vi "data to acc_gyro.vi"(0 "byte array":u8[](array[numeric]), 1 "gyro range (deg/s)":dbl=250.0, 2 "accel range (m/s2)":dbl=8.0) -> (3 "acc gyro data":T1)   [LabVIEW 2012]
uses:
  acc_gyro_data.ctl
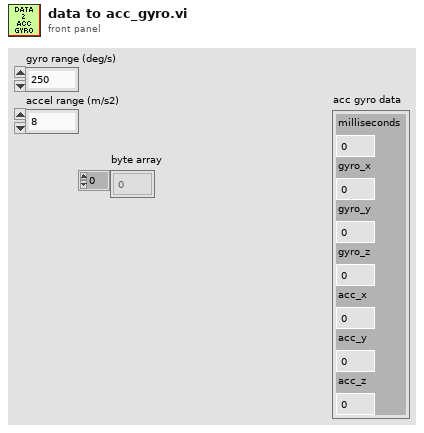
[diagram p1: front panel]
types:
  T1 = typedef "acc_gyro_data.ctl" = cluster{"milliseconds":u64, "gyro_x":dbl, "gyro_y":dbl, "gyro_z":dbl, "acc_x":dbl, "acc_y":dbl, "acc_z":dbl}
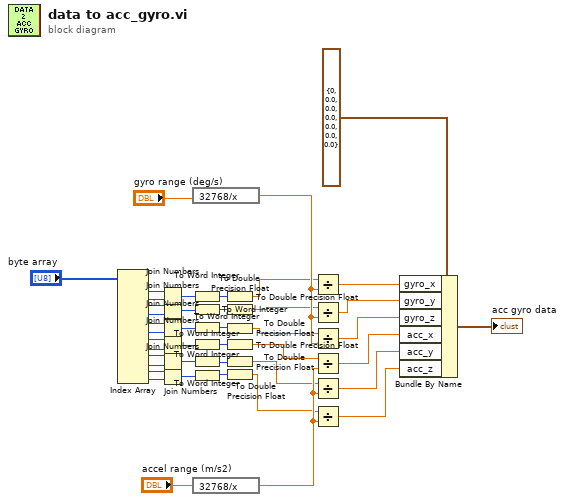
[diagram p0: block diagram]
diagram:
  n1 = Index Array(array="byte array") -> (element #1=w42:u8, element #2=w41:u8, element #3=w40:u8, element #4=w39:u8, element #5=w38:u8, element #6=w37:u8, element #7=w36:u8, element #8=w35:u8, element #9=w34:u8, element #10=w33:u8, element #11=w32:u8, element #12=w31:u8)  [unwired: 12 in]
  n2 = Join Numbers(hi=w42, lo=w41) -> ((hi.lo)=w30:u16)
  n3 = Join Numbers(hi=w40, lo=w39) -> ((hi.lo)=w29:u16)
  n4 = Join Numbers(hi=w38, lo=w37) -> ((hi.lo)=w28:u16)
  n5 = Join Numbers(hi=w36, lo=w35) -> ((hi.lo)=w27:u16)
  n6 = Join Numbers(hi=w34, lo=w33) -> ((hi.lo)=w26:u16)
  n7 = Join Numbers(hi=w32, lo=w31) -> ((hi.lo)=w25:u16)
  n8 = To Word Integer(number=w30) -> (16bit integer=w24:i16)
  n9 = To Word Integer(number=w29) -> (16bit integer=w23:i16)
  n10 = To Word Integer(number=w28) -> (16bit integer=w22:i16)
  n11 = To Word Integer(number=w27) -> (16bit integer=w21:i16)
  n12 = To Word Integer(number=w26) -> (16bit integer=w20:i16)
  n13 = To Word Integer(number=w25) -> (16bit integer=w19:i16)
  n14 = expression code="32768/x"("gyro range (deg/s)") -> (w7:dbl)
  n15 = expression code="32768/x"("accel range (m/s2)") -> (w9:dbl)
  n16 = To Double Precision Float(number=w24) -> (double precision float=w6:dbl)
  n17 = To Double Precision Float(number=w23) -> (double precision float=w5:dbl)
  n18 = To Double Precision Float(number=w22) -> (double precision float=w4:dbl)
  n19 = To Double Precision Float(number=w21) -> (double precision float=w3:dbl)
  n20 = To Double Precision Float(number=w20) -> (double precision float=w2:dbl)
  n21 = To Double Precision Float(number=w19) -> (double precision float=w1:dbl)
  n22 = Divide(x=w6, y=w7) -> (x/y=w18:dbl)
  n23 = Divide(x=w5, y=w7) -> (x/y=w17:dbl)
  n24 = Divide(x=w4, y=w7) -> (x/y=w16:dbl)
  n25 = Divide(x=w3, y=w9) -> (x/y=w15:dbl)
  n26 = Divide(x=w2, y=w9) -> (x/y=w14:dbl)
  n27 = Divide(x=w1, y=w9) -> (x/y=w13:dbl)
  n28 = Bundle By Name(cluster=T1 {"milliseconds"=0, "gyro_x"=0.0, "gyro_y"=0.0, "gyro_z"=0.0, "acc_x"=0.0, "acc_y"=0.0, "acc_z"=0.0} ("acc gyro data 2"), "gyro_x"=w18, "gyro_y"=w17, "gyro_z"=w16, "acc_x"=w15, "acc_y"=w14, "acc_z"=w13) -> (→"acc gyro data":T1)
